vi "StoreMeasurementDataToDB.vi"(0 "UserID":string, 1 "DatabaseConnectionInfo":T1, 2 "Data":dbl[](array[numeric]), 5 "Description":string, 7 "Device ID":string, 9 "Measurement name":string, 11 "error in (no error)":errorcluster, 12 "DataTimestamps":dbl[](array[numeric]), 13 "seconds since 1Jan1904":timestamp) -> (15 "error out":errorcluster)   [LabVIEW 2017]
uses:
  <vilib>/addons/database/Auxilliary.llb/DB Tools Transaction.ctl
  <vilib>/addons/database/Connection.llb/DB Tools Open Connec (Path).vi
  <vilib>/addons/database/Connection.llb/Conn Transaction.vi
  <vilib>/addons/database/Connection.llb/Conn Execute.vi
  <vilib>/addons/database/Recordset.llb/Rec Fetch Recordset Data (R).vi
  <vilib>/addons/database/Recordset.llb/Rec Destroy - Connection.vi
  <vilib>/addons/database/_DB Variant To Data/Database Variant To Data.xnode
  <vilib>/addons/database/NI_Database_API.lvlib
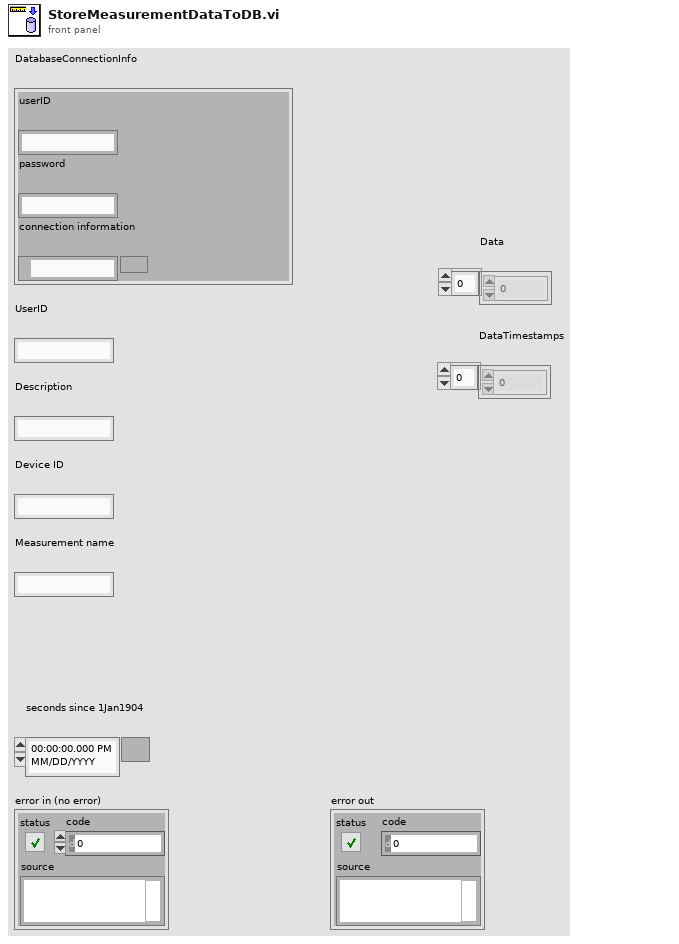
[diagram p1: front panel]
types:
  T1 = cluster{"userID":string, "password":string, "connection information":path}
  T2 = typedef "NI_Database_API.lvlib/DB Tools Transaction.ctl" = enum16{"begin", "commit", "rollback"}
  T3 = typedef "NI_Database_API.lvlib/Conn ObjectReference.ctl" = refnum<k1>
  T4 = typedef "NI_Database_API.lvlib/Rec ObjectReference.ctl" = refnum<k1>
  T5 = cluster{string, "date/time string":string, "Description":string, "Device ID":string, "UserID":string, "Measurement name":string}
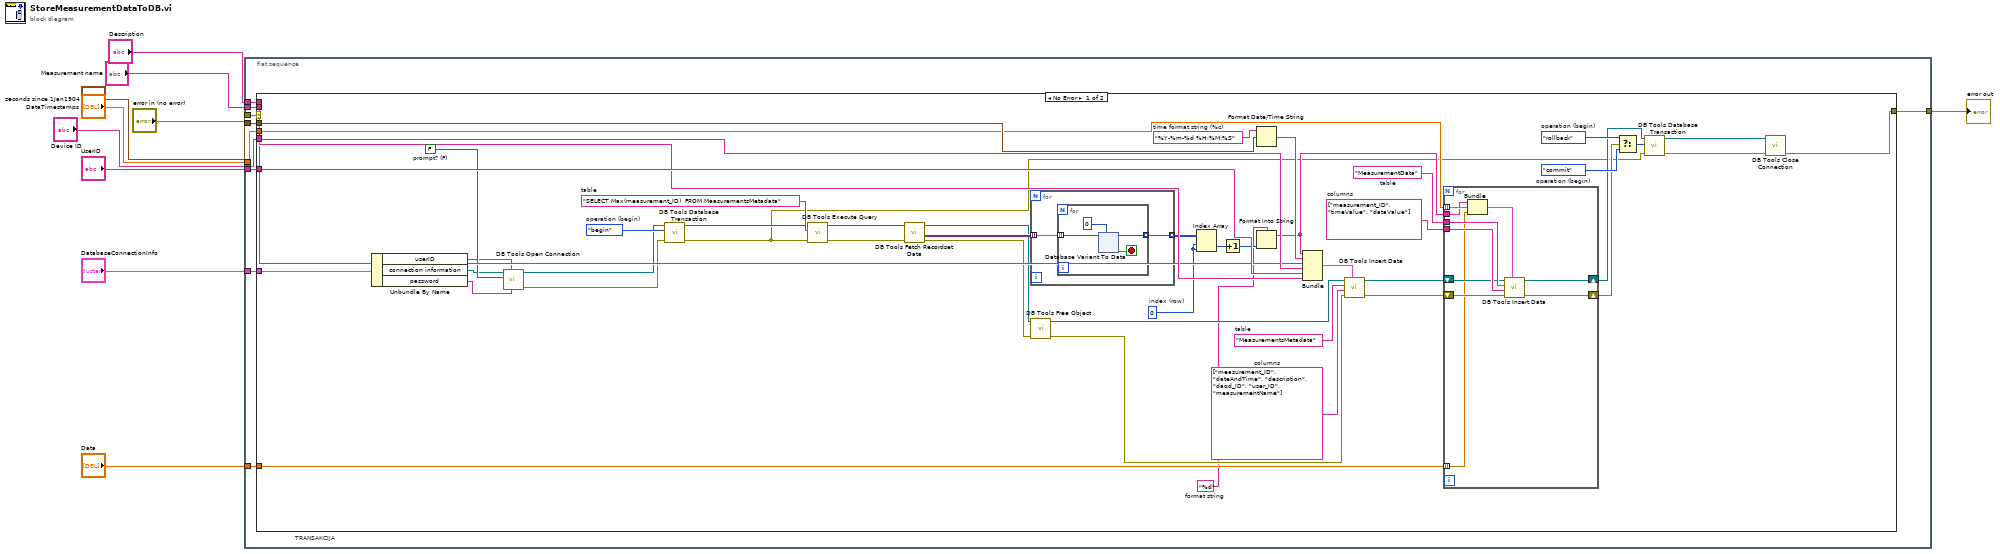
[diagram p0: block diagram]
diagram:
  n1 = flat-sequence {
    tunnel: "DatabaseConnectionInfo" -> [w20]
    tunnel: "seconds since 1Jan1904" -> [w19]
    tunnel: "Device ID" -> [w18]
    tunnel: "UserID" -> [w17]
    tunnel: "error in (no error)" -> [w16]
    tunnel: [w15] -> w6
    tunnel: "DataTimestamps" -> [w14]
    tunnel: "Data" -> [w13]
    tunnel: "Measurement name" -> [w12]
    tunnel: "Description" -> [w11]
    frame #0 {
      # "TRANSAKCIJA"
      n2 = case shown="No Error" w16 {
        selector: w16 -> [_ w117]
        tunnel: [w68 w117] -> w15
        tunnel: w20 -> [w67 _]
        tunnel: w19 -> [w66 _]
        tunnel: w18 -> [w65 _]
        tunnel: w17 -> [w64 _]
        tunnel: w14 -> [w63 _]
        tunnel: w13 -> [w62 _]
        tunnel: w12 -> [w61 _]
        tunnel: w11 -> [w60 _]
        frame No Error {
          w22 = "%d"  # format string
          w30 = 0  # index (row)
          w33 = "SELECT Max(measurement_ID)  FROM MeasurementsMetadata"  # table
          w37 = string[] ["measurement_ID", "timeValue", "dataValue"]  # columns
          w38 = "MeasurementData"  # table
          w46 = DB_Tools_Transaction."rollback"  # operation (begin)
          w47 = DB_Tools_Transaction."commit"  # operation (begin)
          w50 = DB_Tools_Transaction."begin"  # operation (begin)
          w53 = "MeasurementsMetadata"  # table
          w52 = string[] ["measurement_ID", "dateAndTime", "description", "daqd_ID", "user_ID", "measurementName"]  # columns
          w55 = "%Y-%m-%d %H:%M:%S"  # time format string (%c)
          w59 = FALSE  # prompt? (F)
          n3 = Unbundle By Name(w67) -> ("userID"=w58:string, "connection information"=w56:path, "password"=w57:string)
          n4 = call-poly <vilib>:"DB Tools Open Connection.vi"("password"=w57, "userID"=w58, "prompt? (F)"=w59, "connection information"=w56) -> ("error out"=w48:errorcluster, "connection reference"=w49:T3)  [unwired: 4 in]
          n5 = call-poly <vilib>:"DB Tools Database Transaction.vi"("error in (no error)"=w48, "operation (begin)"=w50, "connection reference"=w49) -> ("error out"=w21:errorcluster, "connection reference out"=w27:T3)  [unwired: 3 in]
          n6 = call-poly <vilib>:"DB Tools Execute Query.vi"("error in (no error)"=w21, "SQL query"=w33, "connection reference"=w27) -> ("error out"=w32:errorcluster, "recordset reference"=w34:T4)  [unwired: 5 in]
          n7 = call-poly <vilib>:"DB Tools Fetch Recordset Data.vi"("error in (no error)"=w32, "recordset reference"=w34) -> ("error out"=w26:errorcluster, "recordset data"=w36:variant[][], "recordset reference out"=w35:T4)  [unwired: 3 in]
          n8 = for {
            tunnel: w36 -> [w70] mode=indexing
            tunnel: [w69] -> w31 mode=indexing
            n9 = for {
              tunnel: w70 -> [w74] mode=indexing
              tunnel: [w73] -> w69 mode=indexing
              stop <- w72 stop-if-true
              n10 = xnode "Database Variant To Data"("database variant"=w74, "type"=i64 0) -> ("data"=w73:i64, "error out"=w72:errorcluster)  [unwired: 1 in]
            }
          }
          n11 = call-poly <vilib>:"DB Tools Free Object.vi"("error in (no error)"=w26, "recordset reference"=w35) -> ("error out"=w28:errorcluster, "connection reference"=w29:T3)  [unwired: 8 in]
          n12 = Index Array(array=w31, index (row)=w30, index (col)=w30) -> (element=w25:i64)
          n13 = Increment(x=w25) -> (x+1=w24:i64)
          n14 = Format Date/Time String(time format string (%c)=w55, seconds (now)=w66) -> (date/time string=w54:string)  [unwired: 1 in]
          n15 = Format Into String(format string=w22, w24) -> (resulting string=w23:string)  [unwired: 2 in, 1 out]
          n16 = Bundle(w23, "date/time string"=w54, "Description"=w60, "Device ID"=w65, "UserID"=w64, "Measurement name"=w61) -> (w51:T5)  [unwired: 1 in]
          n17 = call <vilib>:"DB Tools Insert Data.vi"("data"=w51, "error in (no error)"=w28, "columns"=w52, "table"=w53, "connection reference"=w29) -> ("error out"=w41:errorcluster, "connection reference out"=w42:T3)  [unwired: 5 in]
          n18 = for {
            tunnel: w38 -> [w116]
            tunnel: w37 -> [w115]
            shift-right: [w111] -> w40
            shift-left: w42 -> [w114]
            shift-right: [w112] -> w39
            shift-left: w41 -> [w113]
            tunnel: w63 -> [w110] mode=indexing
            tunnel: w62 -> [w109] mode=indexing
            tunnel: w23 -> [w108]
            n19 = Bundle(w108, w110, "number: 0 to 1"=w109) -> (w107:cluster{string, dbl, "number: 0 to 1":dbl})  [unwired: 1 in]
            n20 = call <vilib>:"DB Tools Insert Data.vi"("data"=w107, "error in (no error)"=w113, "columns"=w115, "table"=w116, "connection reference"=w114) -> ("error out"=w112:errorcluster, "connection reference out"=w111:T3)  [unwired: 5 in]
          }
          n21 = Select(t=w46, s=w39, f=w47) -> (s? t:f=w45:T2)
          n22 = call-poly <vilib>:"DB Tools Database Transaction.vi"("error in (no error)"=w21, "operation (begin)"=w45, "connection reference"=w40) -> ("error out"=w43:errorcluster, "connection reference out"=w44:T3)  [unwired: 3 in]
          n23 = call <vilib>:"DB Tools Close Connection.vi"("error in (no error)"=w43, "connection reference"=w44) -> ("error out"=w68:errorcluster)  [unwired: 5 in]
        }
        frame Error {
        }
      }
    }
  }
  "error out" <- w6
